vi "Extend Symbol Path.vi"(3 "Symbol Path":path) -> (1 "Resolved Path":path)   [LabVIEW 2017]
uses:
  <vilib>/Utility/sysdir.llb/System Directory Type.ctl
  <userlib>/_OpenG.lib/file/file.llb/Valid Path - Traditional__ogtk.vi
panel:
  # "#Note [xxx] or <xxx>\n- [application]\n- [desktop]\n- [temp][temporary]\n- [user.lib]\n- [vi.lib]\n-%SystemVariable%, eg: OneDrive"
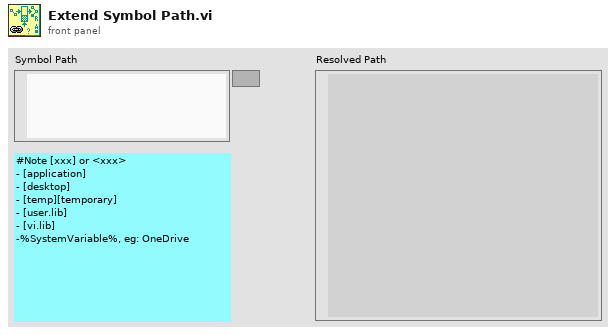
[diagram p1: front panel]
types:
  T1 = enum16{"Absolute path", "Relative path", "<Not A Path>"}
  T2 = typedef "System Directory Type.ctl" = i32
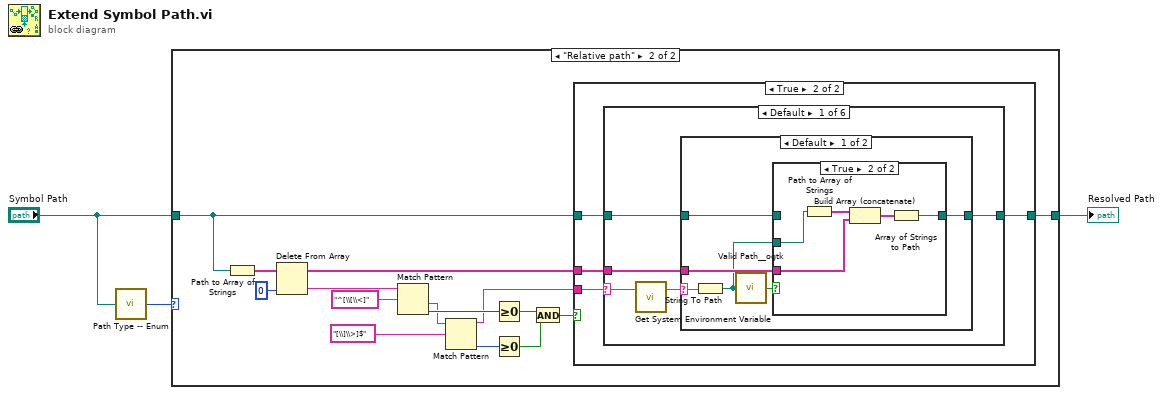
[diagram p0: block diagram]
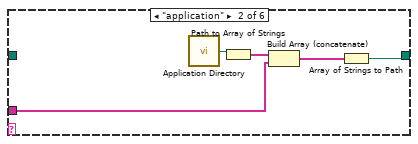
[diagram p6: hidden frame]
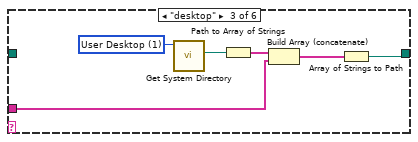
[diagram p7: hidden frame]
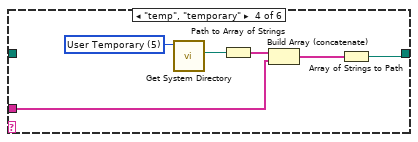
[diagram p8: hidden frame]
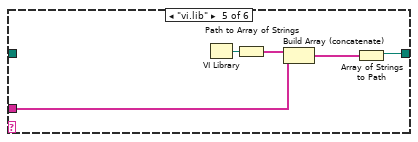
[diagram p9: hidden frame]
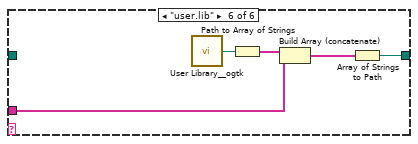
[diagram p10: hidden frame]
diagram:
  n1 = call "Path Type -- Enum.vi"("Value"="Symbol Path") -> ("Enum"=w3:T1)
  n2 = case shown="\"Relative path\"" w3 {
    tunnel: [w4 w11] -> w2
    tunnel: "Symbol Path" -> [w4 w10]
    frame "Absolute path", "<Not A Path>", Default {
    }
    frame "Relative path" {
      n3 = Path to Array of Strings(0:w10) -> (2:w19:string[])  [unwired: 1 out]
      n4 = Delete From Array(array=w19, index=0) -> (deleted portion=w9:string, array with subset deleted=w5:string[])  [unwired: 1 in]
      n5 = Match Pattern(string=w9, regular expression="^[\\[\\<]") -> (after substring=w8:string, offset past match=w16:i32)  [unwired: 1 in, 2 out]
      n6 = Match Pattern(string=w8, regular expression="[\\]\\>]$") -> (before substring=w7:string, offset past match=w15:i32)  [unwired: 1 in, 2 out]
      n7 = Greater Or Equal To 0?(x=w16) -> (x >= 0?=w14:bool)
      n8 = Greater Or Equal To 0?(x=w15) -> (x >= 0?=w13:bool)
      n9 = And(x=w14, y=w13) -> (x .and. y?=w12:bool)
      n10 = case shown="True" w12 {
        tunnel: [w20 w21] -> w11
        tunnel: w10 -> [w20 w23]
        tunnel: w7 -> [_ w24]
        tunnel: w5 -> [_ w22]
        frame False {
        }
        frame True {
          n11 = case shown="Default" w24 {
            selector: w24 -> [w29 _ _ _ _ _]
            tunnel: w23 -> [w26 _ _ _ _ _]
            tunnel: w22 -> [w25 w43 w50 w56 w60 w65]
            tunnel: [w27 w45 w51 w57 w62 w67] -> w21
            frame Default {
              n12 = call "Get System Environment Variable.vi"("Environment Variable Name"=w29) -> ("Value"=w28:string)  [unwired: 2 in]
              n13 = case shown="Default" w28 {
                selector: w28 -> [w35 _]
                tunnel: [w33 w42] -> w27
                tunnel: w26 -> [w32 w42]
                tunnel: w25 -> [w31 _]
                frame Default {
                  n14 = String To Path(string=w35) -> (path=w30:path)
                  n15 = call-poly <userlib>:"Valid Path__ogtk.vi"("path"=w30) -> ("valid"=w34:bool)
                  n16 = case shown="True" w34 {
                    tunnel: [w36 w39] -> w33
                    tunnel: w32 -> [w36 _]
                    tunnel: w31 -> [_ w38]
                    tunnel: w30 -> [_ w37]
                    frame False {
                    }
                    frame True {
                      n17 = Path to Array of Strings(0:w37) -> (2:w40:string[])  [unwired: 1 out]
                      n18 = Build Array (concatenate)(w40, w38) -> (w41:string[])
                      n19 = Array of Strings to Path(0:w41) -> (2:w39:path)  [unwired: 1 in]
                    }
                  }
                }
                frame "" {
                }
              }
            }
            frame "application" {
              n20 = call <vilib>:"Application Directory.vi"() -> ("Application Directory"=w44:path)
              n21 = Path to Array of Strings(0:w44) -> (2:w46:string[])  [unwired: 1 out]
              n22 = Build Array (concatenate)(w46, w43) -> (w47:string[])
              n23 = Array of Strings to Path(0:w47) -> (2:w45:path)  [unwired: 1 in]
            }
            frame "desktop" {
              w49 = T2 1 items=["User Home"=0, "User Desktop"=1, "User Documents"=2, "User Application Data"=3, "User Preferences"=4, "User Temporary"=5, "Public Documents"=6, "Public Application Data"=7, "Public Preferences"=8, "Public Cache"=13, "System Core Libraries"=9, "System Installed Libraries"=10, "Application Files"=11, "Boot Volume Root"=12] ("system directory type")
              n24 = call <vilib>:"Get System Directory.vi"("system directory type"=w49) -> ("system directory"=w48:path)  [unwired: 10 in]
              n25 = Path to Array of Strings(0:w48) -> (2:w52:string[])  [unwired: 1 out]
              n26 = Build Array (concatenate)(w52, w50) -> (w53:string[])
              n27 = Array of Strings to Path(0:w53) -> (2:w51:path)  [unwired: 1 in]
            }
            frame "temp", "temporary" {
              w55 = T2 5 items=["User Home"=0, "User Desktop"=1, "User Documents"=2, "User Application Data"=3, "User Preferences"=4, "User Temporary"=5, "Public Documents"=6, "Public Application Data"=7, "Public Preferences"=8, "Public Cache"=13, "System Core Libraries"=9, "System Installed Libraries"=10, "Application Files"=11, "Boot Volume Root"=12] ("system directory type")
              n28 = call <vilib>:"Get System Directory.vi"("system directory type"=w55) -> ("system directory"=w54:path)  [unwired: 10 in]
              n29 = Path to Array of Strings(0:w54) -> (2:w58:string[])  [unwired: 1 out]
              n30 = Build Array (concatenate)(w58, w56) -> (w59:string[])
              n31 = Array of Strings to Path(0:w59) -> (2:w57:path)  [unwired: 1 in]
            }
            frame "vi.lib" {
              n32 = VI Library() -> (path=w61:path)
              n33 = Path to Array of Strings(0:w61) -> (2:w63:string[])  [unwired: 1 out]
              n34 = Build Array (concatenate)(w63, w60) -> (w64:string[])
              n35 = Array of Strings to Path(0:w64) -> (2:w62:path)  [unwired: 1 in]
            }
            frame "user.lib" {
              n36 = call <userlib>:"User Library__ogtk.vi"() -> ("User Library (+ Relative)"=w66:path)  [unwired: 1 in]
              n37 = Path to Array of Strings(0:w66) -> (2:w68:string[])  [unwired: 1 out]
              n38 = Build Array (concatenate)(w68, w65) -> (w69:string[])
              n39 = Array of Strings to Path(0:w69) -> (2:w67:path)  [unwired: 1 in]
            }
          }
        }
      }
    }
  }
  "Resolved Path" <- w2
